vi "Shut Down Device.vi"(8 "error in (no error)":errorcluster, 11 "TE2000 in":refnum<class "TE2000.lvclass">) -> (0 "error out":errorcluster, 3 "TE2000 out":refnum<class "TE2000.lvclass">)   [LabVIEW 2014, in "TE2000.lvlib" / "TE2000.lvclass"]
uses:
  TE2000.lvclass
  TE2000.lvclass/TE2000.ctl
  Device/Device.lvclass
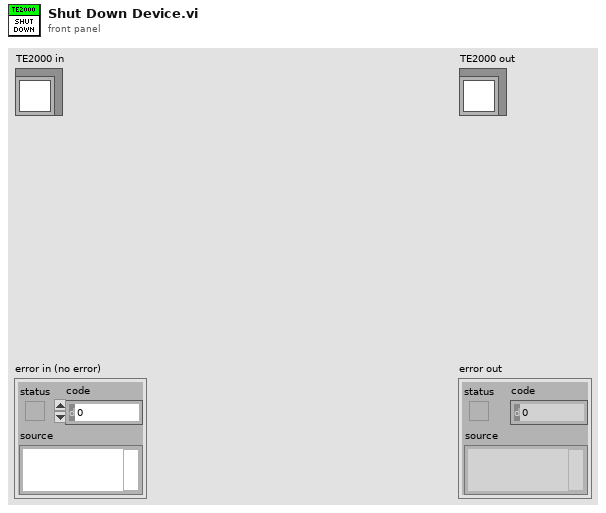
[diagram p1: front panel]
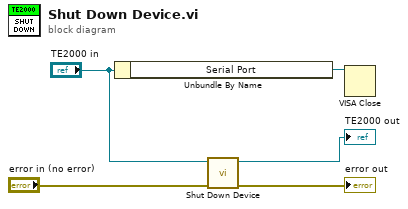
[diagram p0: block diagram]
diagram:
  n1 = Unbundle By Name("TE2000 in") -> ("Serial Port"=w1:refnum<visa-resource-name>)
  n2 = call-parent "Shut Down Device.vi"("error in (no error)"="error in (no error)", "Device in"="TE2000 in") -> ("error out"=→"error out":errorcluster, "Device out"=→"TE2000 out":refnum<class "TE2000.lvclass">)  [unwired: 8 in]
  n3 = VISA Close(VISA resource name=w1) -> ()  [unwired: 1 in, 1 out]
